vi "GenerateTracePlotData.vi"(5 "Reference bead#":i32, 6 "ResultManager":T1, 7 "Subtract reference":bool, 9 "Number of frames to display":i32, 10 "Start frame for trace display":i32, 11 "Bead index":i32) -> (2 "Bead Z":sgl[](array[numeric]), 3 "Bead XY":sgl[][](array[numeric]))   [LabVIEW 2011]
uses:
  qtrk/QTrkLVBinding/ResultManagerInstance.ctl
panel:
  out "Bead Z Waveform":cluster{"index":i32, dbl, sgl[]}
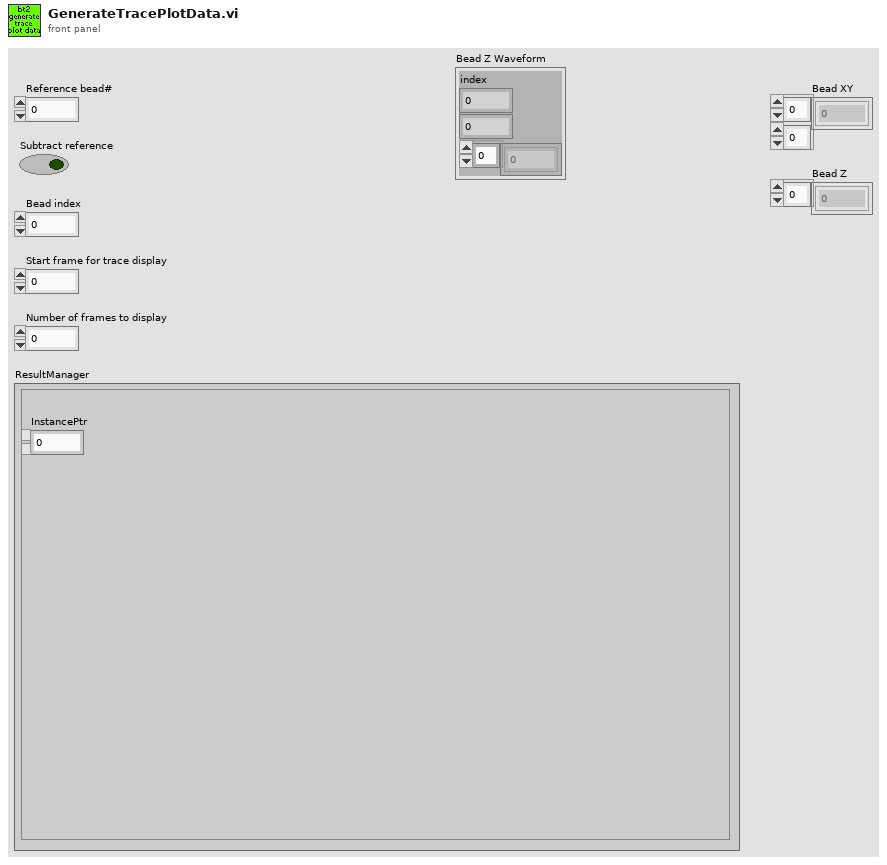
[diagram p1: front panel]
types:
  T1 = typedef "ResultManagerInstance.ctl" = cluster{"InstancePtr":u64}
  T2 = typedef "QTrkLocalizationResult.ctl" = cluster{"Queue Params":T3, "Position":T4, "Fast Estimate Position":cluster{"X":sgl, "Y":sgl}, "Error":i32, "Image mean":sgl}
  T3 = typedef "QTrkLocalizationJob.ctl" = cluster{"Frame#":u32, "Timestamp":u32, "ZLUT Index / bead#":i32, "Initial guess":T4}
  T4 = typedef "XYZf.ctl" = cluster{"X":sgl, "Y":sgl, "Z":sgl}
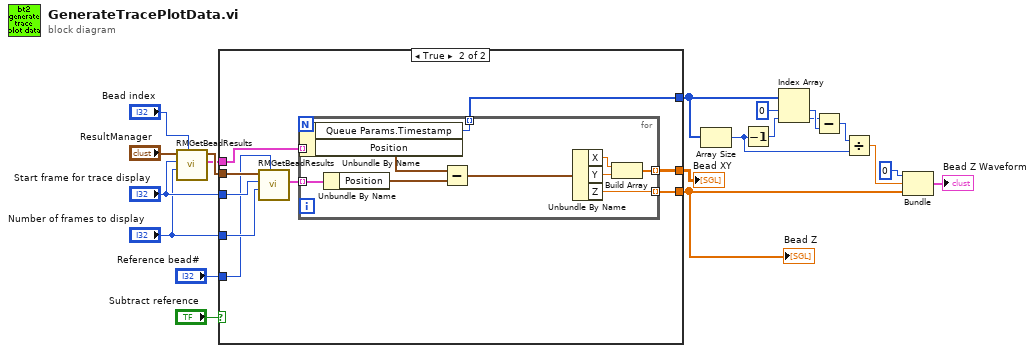
[diagram p0: block diagram]
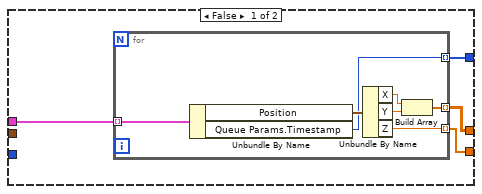
[diagram p2: hidden frame]
diagram:
  n1 = call "RMGetBeadResults.vi"("bead"="Bead index", "numFrames"="Number of frames to display", "startFrame (0)"="Start frame for trace display", "ResultManager"="ResultManager") -> ("results"=w16:T2[], "ResultManager (out)"=w17:T1)  [unwired: 5 in, 1 out]
  n2 = case shown="True" "Subtract reference" {
    tunnel: w17 -> [_ w40]
    tunnel: "Start frame for trace display" -> [_ w39]
    tunnel: "Number of frames to display" -> [_ w38]
    tunnel: w16 -> [w24 w37]
    tunnel: [w23 w35] -> w12
    tunnel: [w22 w34] -> w2
    tunnel: "Reference bead#" -> [_ w33]
    tunnel: [w21 w32] -> w3
    frame False {
      n3 = for {
        tunnel: [w29] -> w23 mode=indexing
        tunnel: [w28] -> w22 mode=indexing
        tunnel: w24 -> [w27] mode=indexing
        tunnel: [w25] -> w21 mode=indexing
        n4 = Unbundle By Name(w27) -> ("Position"=w26:T4, "Queue Params.Timestamp"=w25:u32)
        n5 = Unbundle By Name(w26) -> ("X"=w31:sgl, "Y"=w30:sgl, "Z"=w28:sgl)
        n6 = Build Array(w31, w30) -> (w29:sgl[])
      }
    }
    frame True {
      n7 = call "RMGetBeadResults.vi"("bead"=w33, "numFrames"=w38, "startFrame (0)"=w39, "ResultManager"=w40) -> ("results"=w36:T2[])  [unwired: 5 in, 2 out]
      n8 = for {
        tunnel: w37 -> [w46] mode=indexing
        tunnel: [w48] -> w35 mode=indexing
        tunnel: [w47] -> w34 mode=indexing
        tunnel: w36 -> [w45] mode=indexing
        tunnel: [w41] -> w32 mode=indexing
        n9 = Unbundle By Name(w46) -> ("Queue Params.Timestamp"=w41:u32, "Position"=w44:T4)
        n10 = Unbundle By Name(w45) -> ("Position"=w43:T4)
        n11 = Subtract(x=w44, y=w43) -> (x-y=w42:T4)
        n12 = Unbundle By Name(w42) -> ("X"=w50:sgl, "Y"=w49:sgl, "Z"=w47:sgl)
        n13 = Build Array(w50, w49) -> (w48:sgl[])
      }
    }
  }
  "Bead Z" <- w2
  "Bead XY" <- w12
  n14 = Array Size(array=w3) -> (size(s)=w9:i32)
  n15 = Decrement(x=w9) -> (x-1=w5:i32)
  n16 = Index Array(array=w3, index #1=0 ("index"), index #2=w5) -> (element #1=w7:u32, element #2=w6:u32)
  n17 = Subtract(x=w6, y=w7) -> (x-y=w8:u32)
  n18 = Divide(x=w8, y=w9) -> (x/y=w11:dbl)
  n19 = Bundle("index"=0, w11, w2) -> (→"Bead Z Waveform":cluster{"index":i32, dbl, sgl[]})  [unwired: 1 in]
